vi "SendDashboardData.vi"   [LabVIEW 2018]
uses:
  Global_Var-RefNum/DriversStationData.vi
  <vilib>/Rock Robotics/Network Tables/NT Write Number.vi
  <vilib>/Rock Robotics/Network Tables/NT Write String.vi
  <vilib>/Rock Robotics/Network Tables/NT Write Boolean.vi
types:
  T1 = typedef "ArmTargetPosition.ctl" = enum16{"Forward Cargo Floor Intake", "Forward Cargo Feeder Station", "Forward Cargo Low", "Forward Cargo Middle", "Forward Cargo High", "Forward Cargo CargoShip", "Forward Hatch Floor Intake", "Forward Hatch Feeder Station", "Forward Hatch Low", "Forward Hatch Middle", "Forward Hatch High", "Forward Hatch CargoShip", "Reverse Cargo Floor Intake", "Reverse Cargo Feeder Station", "Reverse Cargo Low", "Reverse Cargo Middle", "Reverse Cargo High", "Reverse Cargo CargoShip", "Reverse Hatch Floor Intake", "Reverse Hatch Feeder Station", "Reverse Hatch Low", "Reverse Hatch Middle", "Reverse Hatch High", "Reverse Hatch CargoShip", "Hold"}
  T2 = typedef "ArmHomingState.ctl" = enum16{"ready", "homing in progress", "homing complete ", "homing failed"}
  T3 = typedef "MPSendState.ctl" = enum16{"Disable", "Commit Points", "Enable", "Done", "Failed"}
  T4 = typedef "MotionProfileControlState.ctl" = enum16{"Manual", "Auto_Idle", "Auto_Run"}
  T5 = typedef "ClimberHomingState.ctl" = enum16{"Ready", "Homing In progress", "Homing Failure", "Homing Success "}
  T6 = typedef "ClimberMode.ctl" = enum16{"Manual", "Auto", "Homing"}
  T7 = typedef "ClimberStates.ctl" = enum16{"Ready ", "Lift Bot ", "Raised Drive", "Raise Front Sticks ", "Raise Back Sticks ", "Park ", "Cancel"}
  T8 = typedef "ArmAbsolutePosition.ctl" = cluster{"X (in)":dbl, "Y (in)":dbl, "Wrist (rad)":dbl}
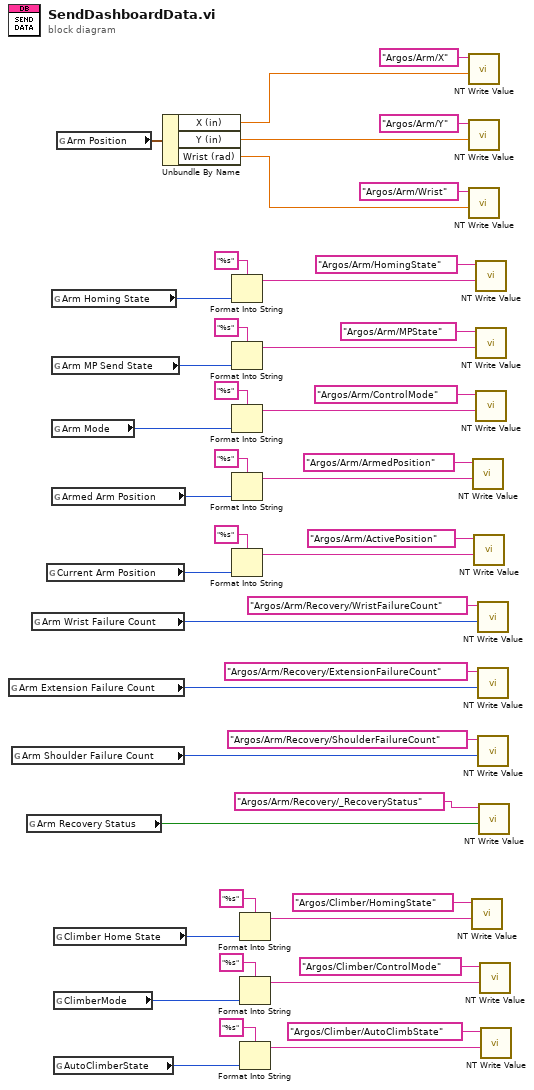
[diagram p0: block diagram]
diagram:
  n1 = global read "DriversStationData.vi" "Arm Extension Failure Count"() -> (w4:u16)
  n2 = global read "DriversStationData.vi" "Arm Shoulder Failure Count"() -> (w3:i16)
  n3 = global read "DriversStationData.vi" "Arm Recovery Status"() -> (w1:bool)
  n4 = global read "DriversStationData.vi" "Arm Wrist Failure Count"() -> (w5:u16)
  n5 = global read "DriversStationData.vi" "Current Arm Position"() -> (w21:T1)
  n6 = global read "DriversStationData.vi" "Arm Homing State"() -> (w40:T2)
  n7 = global read "DriversStationData.vi" "Arm MP Send State"() -> (w24:T3)
  n8 = global read "DriversStationData.vi" "Arm Mode"() -> (w23:T4)
  n9 = global read "DriversStationData.vi" "Armed Arm Position"() -> (w22:T1)
  n10 = global read "DriversStationData.vi" "Climber Home State"() -> (w19:T5)
  n11 = global read "DriversStationData.vi" "ClimberMode"() -> (w15:T6)
  n12 = global read "DriversStationData.vi" "AutoClimberState"() -> (w16:T7)
  n13 = global read "DriversStationData.vi" "Arm Position"() -> (w47:T8)
  n14 = Unbundle By Name(w47) -> ("X (in)"=w44:dbl, "Y (in)"=w45:dbl, "Wrist (rad)"=w46:dbl)
  n15 = Format Into String(format string="%s", w40) -> (resulting string=w37:string)  [unwired: 2 in, 1 out]
  n16 = Format Into String(format string="%s", w24) -> (resulting string=w36:string)  [unwired: 2 in, 1 out]
  n17 = Format Into String(format string="%s", w23) -> (resulting string=w31:string)  [unwired: 2 in, 1 out]
  n18 = Format Into String(format string="%s", w22) -> (resulting string=w30:string)  [unwired: 2 in, 1 out]
  n19 = Format Into String(format string="%s", w21) -> (resulting string=w25:string)  [unwired: 2 in, 1 out]
  n20 = Format Into String(format string="%s", w19) -> (resulting string=w11:string)  [unwired: 2 in, 1 out]
  n21 = Format Into String(format string="%s", w15) -> (resulting string=w10:string)  [unwired: 2 in, 1 out]
  n22 = Format Into String(format string="%s", w16) -> (resulting string=w9:string)  [unwired: 2 in, 1 out]
  n23 = call-poly <vilib>:"NT Write Value.vi"("Numeric"=w44, "Name"="Argos/Arm/X") -> ()  [unwired: 9 in, 1 out]
  n24 = call-poly <vilib>:"NT Write Value.vi"("Numeric"=w45, "Name"="Argos/Arm/Y") -> ()  [unwired: 9 in, 1 out]
  n25 = call-poly <vilib>:"NT Write Value.vi"("Numeric"=w46, "Name"="Argos/Arm/Wrist") -> ()  [unwired: 9 in, 1 out]
  n26 = call-poly <vilib>:"NT Write Value.vi"("String"=w11, "Name"="Argos/Climber/HomingState") -> ()  [unwired: 9 in, 1 out]
  n27 = call-poly <vilib>:"NT Write Value.vi"("String"=w30, "Name"="Argos/Arm/ArmedPosition") -> ()  [unwired: 9 in, 1 out]
  n28 = call-poly <vilib>:"NT Write Value.vi"("String"=w25, "Name"="Argos/Arm/ActivePosition") -> ()  [unwired: 9 in, 1 out]
  n29 = call-poly <vilib>:"NT Write Value.vi"("String"=w37, "Name"="Argos/Arm/HomingState") -> ()  [unwired: 9 in, 1 out]
  n30 = call-poly <vilib>:"NT Write Value.vi"("String"=w36, "Name"="Argos/Arm/MPState") -> ()  [unwired: 9 in, 1 out]
  n31 = call-poly <vilib>:"NT Write Value.vi"("String"=w31, "Name"="Argos/Arm/ControlMode") -> ()  [unwired: 9 in, 1 out]
  n32 = call-poly <vilib>:"NT Write Value.vi"("Numeric"=w5, "Name"="Argos/Arm/Recovery/WristFailureCount") -> ()  [unwired: 9 in, 1 out]
  n33 = call-poly <vilib>:"NT Write Value.vi"("Numeric"=w4, "Name"="Argos/Arm/Recovery/ExtensionFailureCount") -> ()  [unwired: 9 in, 1 out]
  n34 = call-poly <vilib>:"NT Write Value.vi"("Numeric"=w3, "Name"="Argos/Arm/Recovery/ShoulderFailureCount") -> ()  [unwired: 9 in, 1 out]
  n35 = call-poly <vilib>:"NT Write Value.vi"("Boolean"=w1, "Name"="Argos/Arm/Recovery/_RecoveryStatus") -> ()  [unwired: 9 in, 1 out]
  n36 = call-poly <vilib>:"NT Write Value.vi"("String"=w10, "Name"="Argos/Climber/ControlMode") -> ()  [unwired: 9 in, 1 out]
  n37 = call-poly <vilib>:"NT Write Value.vi"("String"=w9, "Name"="Argos/Climber/AutoClimbState") -> ()  [unwired: 9 in, 1 out]
